vi "multi-tau_time.vi"(8 "tau":u32[](array[numeric]), 9 "m":i32=2, 10 "P":i32=64, 11 "No. of shift registers":i32) -> (3 "time multi-tau":ext[](array[numeric]) format="%#_12g")   [LabVIEW 2015]
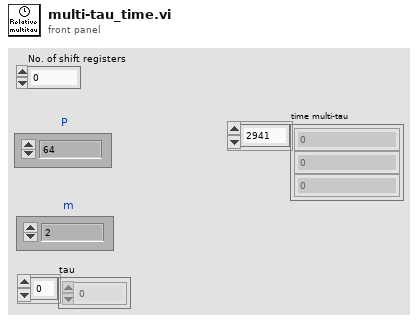
[diagram p1: front panel]
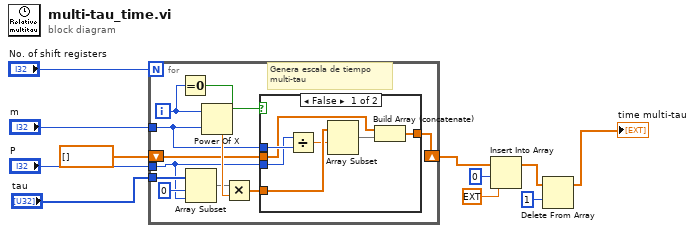
[diagram p0: block diagram]
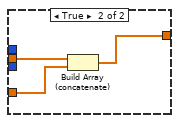
[diagram p2: hidden frame]
diagram:
  n1 = for {
    N: "No. of shift registers" -> [_]
    tunnel: "m" -> [w17]
    tunnel: "tau" -> [w22]
    tunnel: "P" -> [w12]
    shift-right: [w13] -> w2
    shift-left: ext[] [] ("Photon trace A") -> [w15]
    i -> [w18]
    # "Genera escala de tiempo \nmulti-tau"
    n2 = Equal To 0?(x=w18) -> (x = 0?=w19:bool)
    n3 = Array Subset(array=w22, index=0, length=w12) -> (w16:u32[])
    n4 = Power Of X(1:w17, 2:w18) -> (0:w20:dbl)
    n5 = Multiply(x=w16, y=w20) -> (x*y=w14:dbl[])
    n6 = case shown="False" w19 {
      tunnel: [w27 w30] -> w13
      tunnel: w17 -> [w29 _]
      tunnel: w15 -> [w26 w32]
      tunnel: w14 -> [w28 w31]
      tunnel: w12 -> [w24 _]
      frame False {
        n7 = Divide(x=w24, y=w29) -> (x/y=w23:dbl)
        n8 = Array Subset(array=w28, index=w23) -> (w25:dbl[])  [unwired: 1 in]
        n9 = Build Array (concatenate)(w26, w25) -> (w27:ext[])
      }
      frame True {
        n10 = Build Array (concatenate)(w32, w31) -> (w30:ext[])
      }
    }
  }
  n11 = Insert Into Array(array=w2, index=0, new element=ext 0.0 ("new element/subarray")) -> (w4:ext[])
  n12 = Delete From Array(array=w4, length=1) -> (array with subset deleted=→"time multi-tau":ext[])  [unwired: 1 in, 1 out]
